vi "UpdateNetworkImpairment.vi"(8 "ErrorArray In":errorcluster[](array[cluster]), 10 "clBusData In":T1={"BusNumber"=0, "EvtPluginINIFilePath"=path "", "EvtParams"=[], "EvtConfig"={"UTC Time 0"=timestamp(0 s since 1904-01-01), "Nominal Frequency"=60, "Reporting Rate"=60, "Fsamp"=960, "PosSeq"=FALSE}, "Start Time"=0.0, "End Time"=0.0, "PmuImpairPluginINIFilePath"=path "", "PmuImpairParams "=[["960"], ["8.19"], ["164"]], "PmuImpairConfig"={"FilterType"="", "bPosSeq"=TRUE}, "NetImpPluginINIFilePath"=path "", "NetImpParams"=[], "FlagImpPluginINIFilePath"=path "", "FlagImpParams"=[], "EvtReportArray"=[], "EventSignalArray"=[], "ImpairReportArray"=[], "NetworkTime"=[], "PktLoss"=[], "FlagImpArray"=[], "OutputToFilePluginINIFilePath"=path "", "Output File Path"=path "", "clConfigOptions"={"TIME_BASE"=1000000, "STN"="Bus_1", "IDCODE"=0, "rdoPolRect"=enum."Rectangular", "rdoFloatInt"=enum."Float", "PHUNIT"=1000000, "rdoFreqDfreq"=enum."Float", "CHNAM"=["VA", "VB", "VC", "V+", "IA", "IB", "IC", "I+"], "chkCfg2Prefix"=TRUE}, "AppPluginINIFilePath"=path "", "AppConfig"=variant, "AppOutput"=variant} {"clConfigOptions"."PHUNIT" max=16777216 step=1 format="%08d"; "clConfigOptions"."IDCODE" format="%02x"; "clConfigOptions"."TIME_BASE" max=16777216 step=1 format="%08d"; "ImpairReportArray"."Synx" format="%#_4g"; "EvtReportArray"."Synx" format="%#_4g"; "EvtConfig"."Reporting Rate" items=["10 FPS"=10, "12 FPS"=12, "15 FPS"=15, "20 FPS"=20, "25 FPS"=25, "30 FPS"=30, "50 FPS"=50, "60 FPS"=60]; "EvtConfig"."Nominal Frequency" items=["50 Hz"=50, "60 Hz"=60]}, 11 "Bus.lvclass In":refnum<class "Bus.lvclass">) -> (0 "ErrorArray Out":errorcluster[](array[cluster]), 2 "clBusData Out":T1={"BusNumber"=0, "EvtPluginINIFilePath"=path "", "EvtParams"=[], "EvtConfig"={"UTC Time 0"=timestamp(0 s since 1904-01-01), "Nominal Frequency"=60, "Reporting Rate"=60, "Fsamp"=960, "PosSeq"=FALSE}, "Start Time"=0.0, "End Time"=0.0, "PmuImpairPluginINIFilePath"=path "", "PmuImpairParams "=[["960"], ["8.19"], ["164"]], "PmuImpairConfig"={"FilterType"="", "bPosSeq"=TRUE}, "NetImpPluginINIFilePath"=path "", "NetImpParams"=[], "FlagImpPluginINIFilePath"=path "", "FlagImpParams"=[], "EvtReportArray"=[], "EventSignalArray"=[], "ImpairReportArray"=[], "NetworkTime"=[], "PktLoss"=[], "FlagImpArray"=[], "OutputToFilePluginINIFilePath"=path "", "Output File Path"=path "", "clConfigOptions"={"TIME_BASE"=1000000, "STN"="Bus_1", "IDCODE"=0, "rdoPolRect"=enum."Rectangular", "rdoFloatInt"=enum."Float", "PHUNIT"=1000000, "rdoFreqDfreq"=enum."Float", "CHNAM"=["VA", "VB", "VC", "V+", "IA", "IB", "IC", "I+"], "chkCfg2Prefix"=TRUE}, "AppPluginINIFilePath"=path "", "AppConfig"=variant, "AppOutput"=variant} {"clConfigOptions"."PHUNIT" max=16777216 step=1 format="%08d"; "clConfigOptions"."IDCODE" format="%02x"; "clConfigOptions"."TIME_BASE" max=16777216 step=1 format="%08d"; "ImpairReportArray"."Synx" format="%#_4g"; "EvtReportArray"."Synx" format="%#_4g"; "EvtConfig"."Reporting Rate" items=["10 FPS"=10, "12 FPS"=12, "15 FPS"=15, "20 FPS"=20, "25 FPS"=25, "30 FPS"=30, "50 FPS"=50, "60 FPS"=60]; "EvtConfig"."Nominal Frequency" items=["50 Hz"=50, "60 Hz"=60]}, 3 "Bus.lvclass Out":refnum<class "Bus.lvclass">)   [LabVIEW 2017, in "Bus_class.lvlib" / "Bus.lvclass"]
uses:
  Bus.lvclass
  TypeDefs/clBusData.ctl
  FrontPanel/TypeDefs/clEventConfig.ctl
  Modules/PmuImpairPlugins/PmuImpairPluginBase_class/TypeDefs/clImpairConfig.ctl
  Modules/EventPlugins/EventPluginBaseClass/TypeDefs/clEvtReportArray.ctl
  Modules/EventPlugins/EventPluginBaseClass/TypeDefs/clEvtReport.ctl
  Modules/EventPlugins/EventPluginBaseClass/TypeDefs/dblEvtSignalArray.ctl
  Modules/NetworkImpairmentModule/PublicAPI/Arguments/Broadcasts/dblNetworkTime.ctl
  Modules/NetworkImpairmentModule/PublicAPI/Arguments/Broadcasts/dblPktLoss.ctl
  Modules/FlagImpairModule/PublicAPI/Arguments/Broadcasts/ui32FlagImpairmentArray.ctl
  Modules/OutputToFilePlugins/OutputToFileBasePlugin/Typedefs/PmuCfgOpt.ctl
  Framework.lvlib
  Modules/EventPlugins/EventPluginBaseClass/EventPluginBaseClass.lvclass
  Modules/NetworkImpairmentModule/NetworkImpairmentModule.lvlib
  Modules/FlagImpairModule/FlagImpairModule.lvlib
  Modules/OutputToFilePlugins/OutputToFileBasePlugin/OutputToFileBasePlugin.lvclass
  Modules/PmuImpairPlugins/PmuImpairPluginBase_class/PmuImpairPluginBase.lvclass
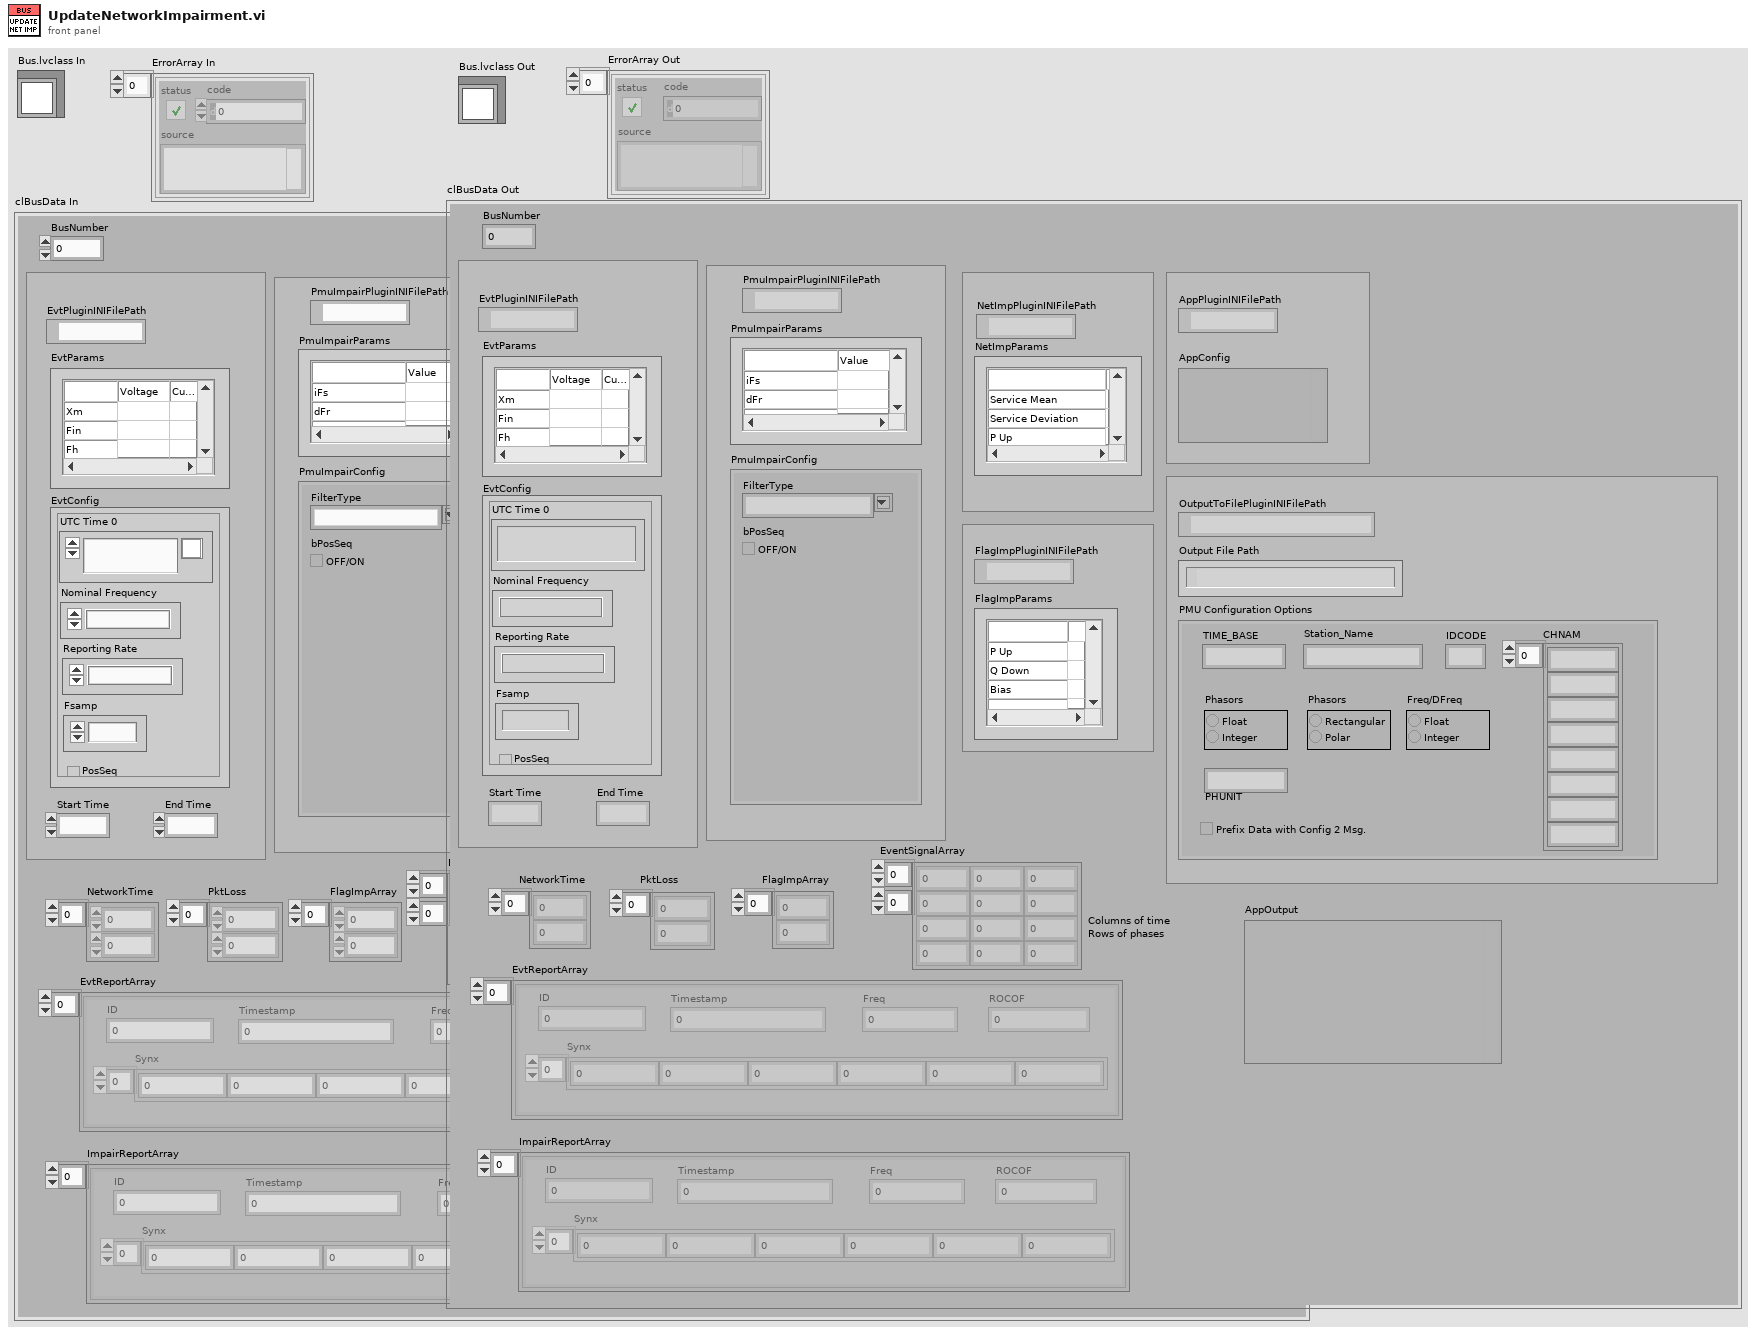
[diagram p1: front panel]
types:
  T1 = typedef "Bus_class.lvlib/Bus.lvclass/clBusData.ctl" = cluster{"BusNumber":u8, "EvtPluginINIFilePath":path, "EvtParams":string[][], "EvtConfig":T2, "Start Time":dbl, "End Time":dbl, "PmuImpairPluginINIFilePath":path, "PmuImpairParams ":string[][], "PmuImpairConfig":T3, "NetImpPluginINIFilePath":path, "NetImpParams":string[][], "FlagImpPluginINIFilePath":path, "FlagImpParams":string[][], "EvtReportArray":T4, "EventSignalArray":T6, "ImpairReportArray":T4, "NetworkTime":T7, "PktLoss":T8, "FlagImpArray":T9, "OutputToFilePluginINIFilePath":path, "Output File Path":path, "clConfigOptions":T10, "AppPluginINIFilePath":path, "AppConfig":variant, "AppOutput":variant}
  T2 = typedef "Framework.lvlib/clEventConfig.ctl" = cluster{"UTC Time 0":timestamp, "Nominal Frequency":u16, "Reporting Rate":u16, "Fsamp":u32, "PosSeq":bool}
  T3 = typedef "PmuImpairPlugins.lvlib/PmuImpairPluginBase.lvclass/clImpairConfig.ctl" = cluster{"FilterType":string, "bPosSeq":bool}
  T4 = typedef "EventPlugins.lvlib/EventPluginBaseClass.lvclass/clEvtReportArray.ctl" = T5[]
  T5 = typedef "EventPlugins.lvlib/EventPluginBaseClass.lvclass/clEvtReport.ctl" = cluster{"Timestamp":dbl, "Synx":cdb[], "Freq":dbl, "ROCOF":dbl, "ID":i16}
  T6 = typedef "EventPlugins.lvlib/EventPluginBaseClass.lvclass/dblEvtSignalArray.ctl" = dbl[][]
  T7 = typedef "NetworkImpairmentModule.lvlib/dblNetworkTime.ctl" = dbl[]
  T8 = typedef "NetworkImpairmentModule.lvlib/dblPktLoss.ctl" = dbl[]
  T9 = typedef "FlagImpairModule.lvlib/ui32FlagImpairmentArray.ctl" = u32[]
  T10 = typedef "OutputToFilePlugins.lvlib/OutputToFileBasePlugin.lvclass/PmuCfgOpt.ctl" = cluster{"TIME_BASE":u64, "STN":string, "IDCODE":u16, "rdoPolRect":enum32{"Rectangular", "Polar"}, "rdoFloatInt":enum32{"Float", "Integer"}, "PHUNIT":u64, "rdoFreqDfreq":enum32{"Float", "Integer"}, "CHNAM":string[], "chkCfg2Prefix":bool}
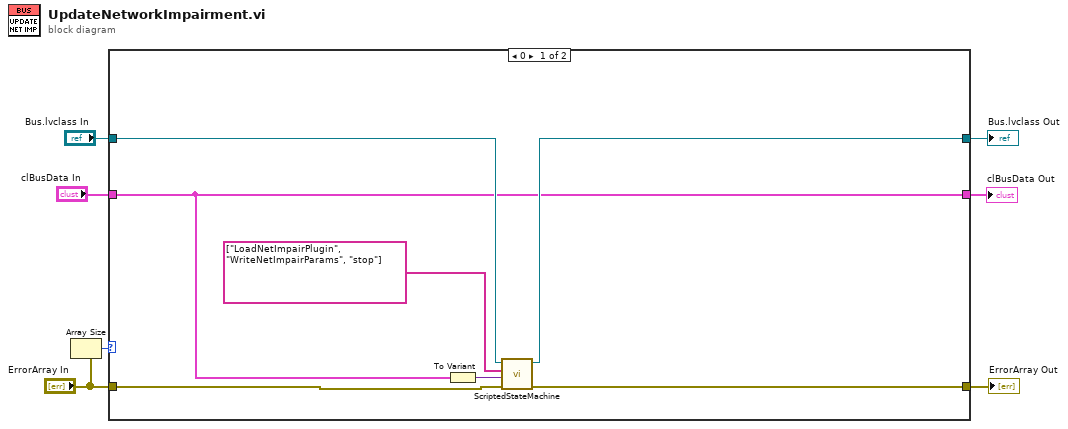
[diagram p0: block diagram]
diagram:
  n1 = Array Size(array="ErrorArray In") -> (size(s)=w6:i32)
  n2 = case shown="0" w6 {
    tunnel: [w14 w17] -> w7
    tunnel: "ErrorArray In" -> [w12 w17]
    tunnel: "Bus.lvclass In" -> [w13 w16]
    tunnel: [w11 w16] -> w3
    tunnel: "clBusData In" -> [w10 w15]
    tunnel: [w10 w15] -> w1
    frame 0 {
      n3 = To Variant(anything=w10) -> (Variant=w9:variant)
      n4 = call "ScriptedStateMachine.vi"("ErrorArray In"=w12, "Data in"=w9, "Script"=string[] ["LoadNetImpairPlugin", "WriteNetImpairParams", "stop"], "Bus"=w13) -> ("ErrorArray Out"=w14:errorcluster[], "Bus"=w11:refnum<class "Bus.lvclass">)  [unwired: 5 in, 1 out]
    }
    frame 1, Default {
    }
  }
  "ErrorArray Out" <- w7
  "Bus.lvclass Out" <- w3
  "clBusData Out" <- w1
